vi "Runtest Queue Handler.vi"(0 "Runtest Queue":refnum<queue>) -> ()   [LabVIEW 2011]
uses:
  www/cgi-bin/runtest/runtest Queue.ctl
  www/tests/Test Output.ctl
  database/Fields/Field Record.ctl
  database/Fields/Field DataTypes.ctl
  database/Fields/Field NextItem.ctl
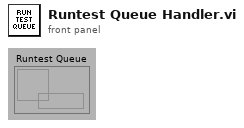
[diagram p1: front panel]
types:
  T1 = typedef "runtest Queue.ctl" = cluster{"Test Output":T2, "Overwrite Existing?":bool, "Print?":bool, "sTestId":string, "Test Station IP (\"\")":string, "sxUsername (\"\")":string, "sDatasheetsCSV (\"\")":string, "Fields":T3[]}
  T2 = typedef "Test Output.ctl" = cluster{"Status":string, "Message":string, "Results":string, "Abort All":bool, "Save Results?":bool, "Timing Metrics":string}
  T3 = typedef "Field Record.ctl" = cluster{"ixField":i32, "iSequenceOrder":i32, "sxFieldId":string, "sxSequenceId":string, "sDisplayName":string, "sValue":string, "sUnits":string, "nDataType":T4, "nNextItem":T5, "fSystem":bool, "fSystemValue":bool, "fRequired":bool, "fSetAtTest":bool, "fTestField":bool, "fDeleted":bool, "fIndexed":bool, "fFreeList":bool}
  T4 = typedef "Field DataTypes.ctl" = enum32{"text", "numeric", "list", "timestamp", "boolean"}
  T5 = typedef "Field NextItem.ctl" = enum32{"Reset", "Retain", "Auto-Increment"}
  T6 = typedef "Connection Refnum.ctl" = cluster{"Environment Handle":i32, "Connection Handle":i32}
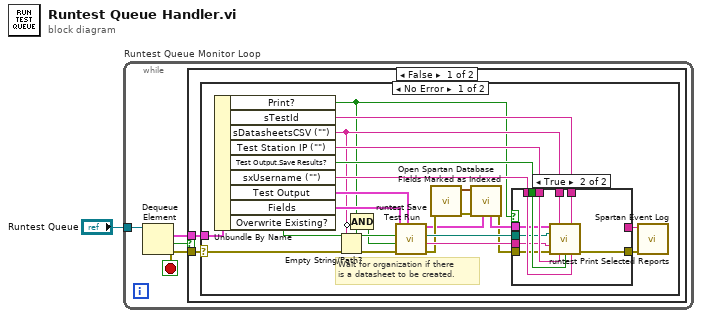
[diagram p0: block diagram]
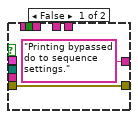
[diagram p2: hidden frame]
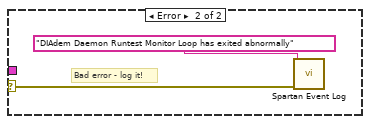
[diagram p3: hidden frame]
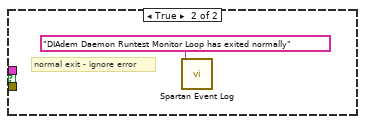
[diagram p4: hidden frame]
diagram:
  n1 = while "Runtest Queue Monitor Loop" {
    tunnel: "Runtest Queue" -> [w5]
    stop <- w2 stop-if-true
    n2 = Dequeue Element(queue=w5) -> (element=w4:T1, timed out?=w3:bool, error out=w2:errorcluster)  [unwired: 1 in, 2 out]
    n3 = case shown="False" w3 {
      tunnel: w4 -> [w7 _]
      tunnel: w2 -> [w6 _]
      frame False {
        n4 = case shown="No Error" w6 {
          selector: w6 -> [w26 w43]
          tunnel: w7 -> [w18 _]
          frame No Error {
            # "Wait for organization if there\nis a datasheet to be created."
            n5 = Unbundle By Name(w18) -> ("Print?"=w9:bool, "sTestId"=w30:string, "sDatasheetsCSV (\"\")"=w12:string, "Test Station IP (\"\")"=w27:string, "Test Output.Save Results?"=w28:bool, "sxUsername (\"\")"=w29:string, "Test Output"=w25:T2, "Fields"=w24:T3[], "Overwrite Existing?"=w23:bool)
            n6 = Empty String/Path?(string/path=w12) -> (empty?=w10:bool)
            n7 = Compound Arithmetic op=AND(w9, invert w10) -> (w8:bool)
            n8 = call "runtest Save Test Run.vi"("Test Output"=w25, "error in (no error)"=w26, "Wait for Organization? (f)"=w8, "Overwrite Existing? (f)"=w23, "Fields In"=w24) -> ("error out"=w20:errorcluster, "Run ID String"=w21:string, "Data File Path"=w22:path, "Fields Out"=w19:T3[])  [unwired: 3 out]
            n9 = call "Open Spartan Database.vi"("error in (no error)"=w20) -> ("error out"=w16:errorcluster, "Connection Refnum"=w15:T6)  [unwired: 9 in]
            n10 = call "Fields Marked as Indexed.vi"("Fields In"=w19, "error in (no error)"=w16, "Connection Refnum"=w15) -> ("error out"=w13:errorcluster, "Fields Out"=w14:T3[])  [unwired: 7 out]
            n11 = case shown="True" w9 {
              tunnel: w30 -> [_ w42]
              tunnel: w29 -> [_ w41]
              tunnel: w28 -> [_ w40]
              tunnel: w27 -> [_ w39]
              tunnel: w22 -> [_ w38]
              tunnel: w21 -> [_ w37]
              tunnel: [w32 w36] -> w17
              tunnel: w14 -> [_ w35]
              tunnel: w13 -> [w32 w34]
              tunnel: w12 -> [_ w33]
              tunnel: ["Printing bypassed do to sequence settings." ("message (\"\")") _] -> w11
              frame False {
              }
              frame True {
                n12 = call "runtest Print Selected Reports.vi"("Fields"=w35, "sDatasheetsCSV (\"\")"=w33, "sTestId"=w42, "Data File Path"=w38, "Run ID String (\"\")"=w37, "error in (no error)"=w34, "Test Station IP (\"\")"=w39, "Save Results?"=w40, "sxUsername (\"\")"=w41) -> ("error out"=w36:errorcluster)  [unwired: 6 in]
              }
            }
            n13 = call "Spartan Event Log.vi"("error in (no error)"=w17, "message (\"\")"=w11) -> ()  [unwired: 3 in, 4 out]
          }
          frame Error {
            # "Bad error - log it!"
            n14 = call "Spartan Event Log.vi"("error in (no error)"=w43, "message (\"\")"="DIAdem Daemon Runtest Monitor Loop has exited abnormally" ("name (unnamed)")) -> ()  [unwired: 3 in, 4 out]
          }
        }
      }
      frame True {
        # "normal exit - ignore error"
        n15 = call "Spartan Event Log.vi"("message (\"\")"="DIAdem Daemon Runtest Monitor Loop has exited normally" ("message (\"\")")) -> ()  [unwired: 4 in, 4 out]
      }
    }
  }
